vi "Event FGV.vi"(7 "Event FGV Actions":T1, 8 "error in":errorcluster) -> (0 "error out":errorcluster, 2 "Event Registration Refnum":refnum<event-registration>, 3 "API Event Message":refnum<user-event>)   [LabVIEW 2020, in "GUI.lvlib"]
doc: "Handle message queue reference operations for this component.\n\n<b>Create</b> - Obtain a message queue reference and store it in a Feedback Node.\n<b>Get</b> - Retrieve a previously stored message queue reference from the Feedback Node.\n<b>Destroy</b> - Destroy the stored message queue reference."
uses:
  GUI.lvlib
  Event FGV Actions.ctl
  Event Type.ctl
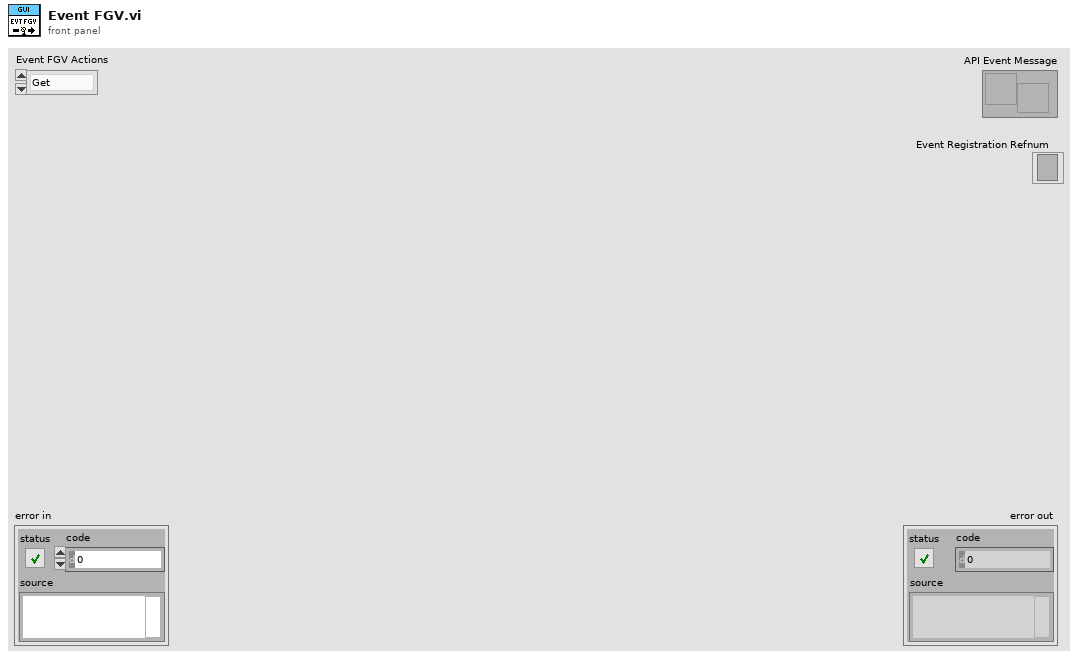
[diagram p1: front panel]
types:
  T1 = typedef "GUI.lvlib/Event FGV Actions.ctl" = enum16{"Get", "Create", "Destroy"}
  T2 = typedef "GUI.lvlib/Event Type.ctl" = cluster{"Command":string, "Payload":variant}
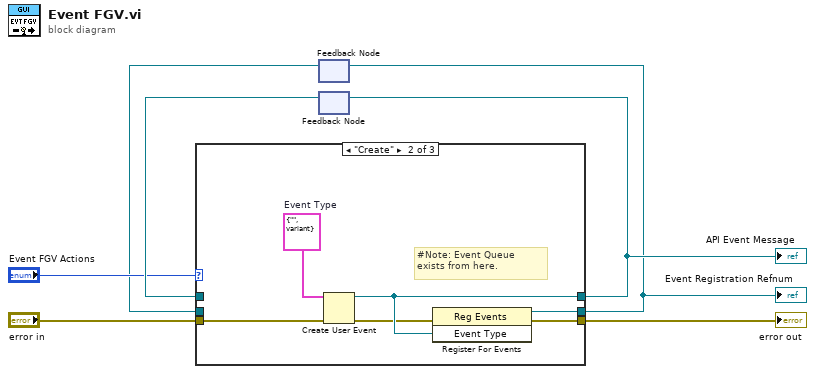
[diagram p0: block diagram]
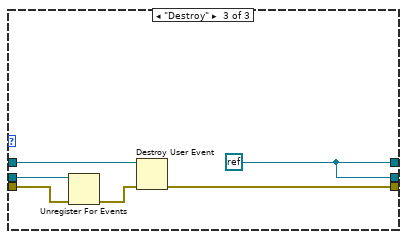
[diagram p3: hidden frame]
diagram:
  n1 = feedback #1() -> (w1:refnum<event-registration>)  [unwired: 1 in]
  n2 = feedback #2() -> (w4:refnum<user-event>)  [unwired: 1 in]
  n3 = case shown="\"Create\"" "Event FGV Actions" {
    tunnel: [w9 w12 w22] -> w7
    tunnel: "error in" -> [w9 w16 w18]
    tunnel: [w10 w14 w20] -> w5
    tunnel: w4 -> [w10 _ w21]
    tunnel: [w8 w11 w20] -> w2
    tunnel: w1 -> [w8 _ w19]
    frame "Get", Default {
    }
    frame "Create" {
      w15 = T2 {"Command"="", "Payload"=variant}  # Event Type
      # "#Note: Event Queue exists from here."
      n4 = Create User Event(user event datatype=w15, error in=w16) -> (user event=w14:refnum<user-event>, error out=w13:errorcluster)
      n5 = register-events(error in=w13, w14) -> (reference out=w11:refnum<event-registration>, error out=w12:errorcluster)  [unwired: 1 in]
    }
    frame "Destroy" {
      w20 = refnum<k0> refnum
      n6 = Unregister For Events(event registration refnum=w19, error in=w18) -> (error out=w17:errorcluster)
      n7 = Destroy User Event(user event=w21, error in=w17) -> (error out=w22:errorcluster)
    }
  }
  "error out" <- w7
  "API Event Message" <- w5
  "Event Registration Refnum" <- w2
  n8 = feedback-in #1(w2) -> ()
  n9 = feedback-in #2(w5) -> ()
